vi "Nested.vi"(8 "Alias":string, 9 "Priority?":bool, 10 "Msg":refnum<class "Msg.lvclass">, 11 "jettl Queue Actor in":refnum<class "jettl Queue Actor.lvclass">) -> (3 "jettl Queue Actor out":refnum<class "jettl Queue Actor.lvclass">)   [LabVIEW 2021, in "jettl.lvlib" / "jettl Queue Actor.lvlib" / "jettl Queue Actor.lvclass"]
uses:
  jettl Queue Actor.lvclass
  Actor/Msg/Msg.lvclass
  jettl Queue Actor.lvclass/jettl Queue Actor.ctl
  jettl.lvlib
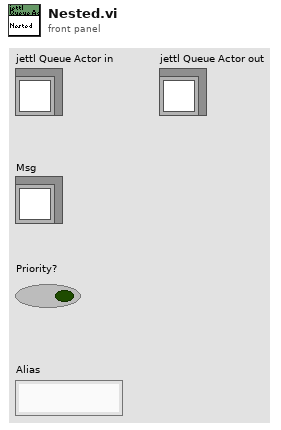
[diagram p1: front panel]
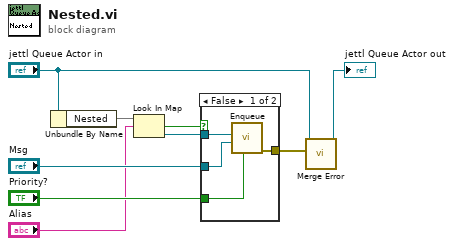
[diagram p0: block diagram]
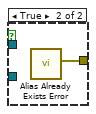
[diagram p2: hidden frame]
diagram:
  n1 = Unbundle By Name("jettl Queue Actor in") -> ("Nested"=w5:map{string, refnum<data-value>})
  n2 = Look In Map(map=w5, key="Alias") -> (key not found?=w4:bool, value=w7:refnum<data-value>)  [unwired: 1 in]
  n3 = case shown="False" w4 {
    tunnel: [w13 w14] -> w1
    tunnel: "Priority?" -> [w12 _]
    tunnel: "Msg" -> [w11 _]
    tunnel: w7 -> [w10 _]
    frame False {
      n4 = call "Enqueue.vi"("Priority?"=w12, "Msg"=w11, "Queue"=w10) -> ("error out"=w13:errorcluster)  [unwired: 8 in]
    }
    frame True {
      n5 = call "Alias Already Exists Error.vi"() -> ("Error"=w14:errorcluster)  [unwired: 11 in]
    }
  }
  n6 = call-dynamic "Merge Error.vi"("Error"=w1, "jettl Queue Actor in"="jettl Queue Actor in") -> ("jettl Queue Actor out"=→"jettl Queue Actor out":refnum<class "jettl Queue Actor.lvclass">)  [unwired: 9 in]
